vi "I2C Read Float.vi"(6 "error in (no error)":errorcluster, 9 "I2CDevRef in":T1 {"Device Address" format="%.0x"}) -> (0 "error out":errorcluster, 2 "value":sgl, 3 "I2CDevRef out":T1 {"Device Address" format="%.0x"})   [LabVIEW 2014]
uses:
  <vilib>/Rock Robotics/WPI/I2C/WPI_I2CDevRef.ctl
  <vilib>/Rock Robotics/SystemInterfaces/Typedef/FPGA_TypedefDigitalModule.ctl
  <vilib>/Rock Robotics/SystemInterfaces/i2clib/i2c_bus.ctl
panel:
  out "Data Out":u8[](array[numeric])
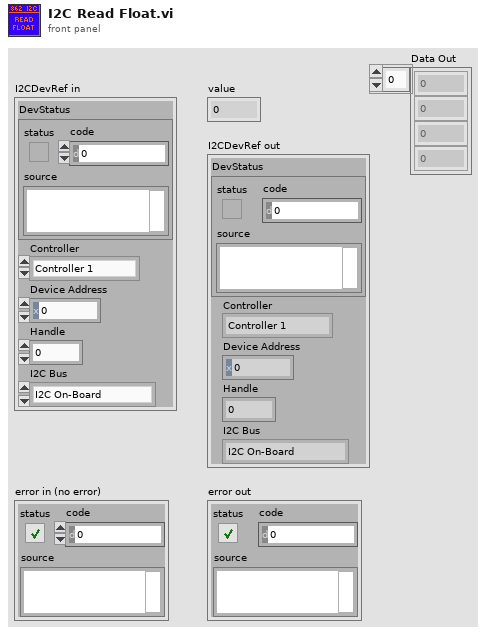
[diagram p1: front panel]
types:
  T1 = typedef "WPI_I2CDevRef.ctl" = cluster{"DevStatus":errorcluster, "Controller":T2, "Device Address":u8, "Handle":i32, "I2C Bus":T3}
  T2 = typedef "FPGA_TypedefDigitalModule.ctl" = enum16{"Controller 1"}
  T3 = typedef "i2c_bus.ctl" = enum16{"I2C On-Board", "I2C MXP", "Invalid"}
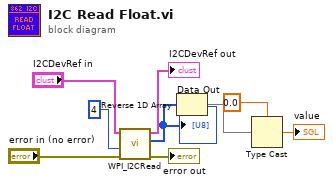
[diagram p0: block diagram]
diagram:
  n1 = call <vilib>:"WPI_I2CRead.vi"("error in (no error)"="error in (no error)", "I2CBytesToRead"=u8 4, "I2CDevRef"="I2CDevRef in") -> ("error out"=→"error out":errorcluster, "Data Out"=w3:u8[], "I2CDevRef"=→"I2CDevRef out":T1)  [unwired: 6 in]
  "Data Out" <- w3
  n2 = Reverse 1D Array(array=w3) -> (reversed array=w4:u8[])
  n3 = Type Cast(type=sgl 0.0 ("number"), x=w4) -> (*(type *) &x=→"value":sgl)
